vi "resize U16 2D img (SubVI).vi"(7 "Interpolation Type":u32(ring)=1 items=["Zero Order", "Bi-Linear", "Quadratic", "Cubic Spline"], 8 "IMAQ(T)/1D-indexing(1F)":bool=TRUE, 9 "Y Resolution":i32, 10 "X Resolution":i32, 11 "Array":u16[][](array[numeric])) -> (3 "Image Pixels (U16)":u16[][](array[numeric]))   [LabVIEW 2024]
uses:
  <vilib>/vision/NI_Vision_Development_Module.lvlib
panel:
  out "time":dbl
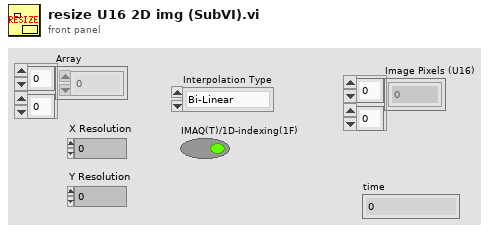
[diagram p1: front panel]
types:
  T1 = typedef "Image Type" = u32
  T2 = typedef "IMAQ Image.ctl" = refnum<image>
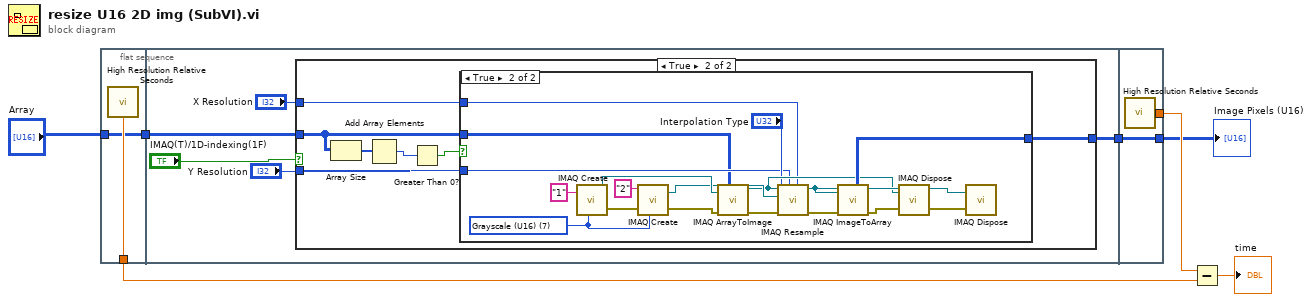
[diagram p0: block diagram]
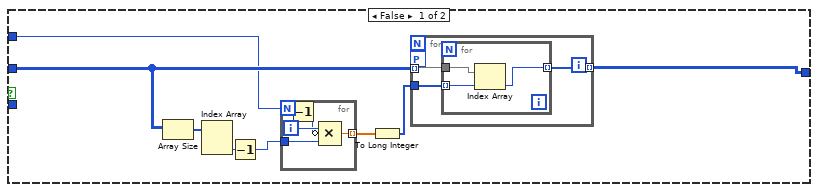
[diagram p2: hidden frame]
diagram:
  n1 = flat-sequence {
    tunnel: [w9] -> w6
    tunnel: [w8] -> w5
    tunnel: "Array" -> [w8]
    tunnel: w5 -> [w13]
    tunnel: [w14] -> w2
    tunnel: [w61] -> w7
    tunnel: [w60] -> w3
    tunnel: w2 -> [w60]
    frame #0 {
      n2 = call <vilib>:"High Resolution Relative Seconds.vi"() -> ("relative seconds"=w9:dbl)
    }
    frame #1 {
      n3 = case shown="True" "IMAQ(T)/1D-indexing(1F)" {
        tunnel: [w22 w40] -> w14
        tunnel: w13 -> [w21 w35]
        tunnel: "X Resolution" -> [w15 w39]
        tunnel: "Y Resolution" -> [_ w38]
        frame False {
          n4 = Array Size(array=w21) -> (size(s)=w20:i32[])
          n5 = Index Array(array=w20) -> (element #2=w19:i32)  [unwired: 2 in, 1 out]
          n6 = Decrement(x=w19) -> (x-1=w17:i32)
          n7 = for {
            N: w15 -> [w25]
            tunnel: w17 -> [w26]
            tunnel: [w24] -> w18 mode=indexing
            i -> [w27]
            n8 = Decrement(x=w25) -> (x-1=w23:i32)
            n9 = Compound Arithmetic op=MULTIPLY(w27, invert w23, w26) -> (w24:dbl)
          }
          n10 = To Long Integer(number=w18) -> (32bit integer=w16:i32[])
          n11 = for {
            tunnel: w21 -> [w30] mode=indexing
            tunnel: [w29] -> w22 mode=indexing
            tunnel: w16 -> [w28]
            workers-P: _ -> [_]
            n12 = for {
              tunnel: w30 -> [w33]
              tunnel: [w32] -> w29 mode=indexing
              tunnel: w28 -> [w31] mode=indexing
              n13 = Index Array(array=w33, index=w31) -> (element=w32:u16)
            }
          }
        }
        frame True {
          n14 = Array Size(array=w35) -> (size(s)=w36:i32[])
          n15 = Add Array Elements(numeric array=w36) -> (sum=w37:i32)
          n16 = Greater Than 0?(x=w37) -> (x > 0?=w34:bool)
          n17 = case shown="True" w34 {
            tunnel: [w41 w49] -> w40
            tunnel: w39 -> [_ w44]
            tunnel: w38 -> [_ w43]
            tunnel: w35 -> [w41 w42]
            frame False {
            }
            frame True {
              w46 = T1 7 items=["Grayscale (U8)", "Grayscale (I16)", "Grayscale (SGL)", "Complex (CSG)", "RGB (U32)", "HSL (U32)", "RGB (U64)", "Grayscale (U16)"] ("Image Type")
              n18 = call "IMAQ Create"("Image Name"="1", "Image Type"=w46) -> ("New Image"=w51:T2, "error out"=w59:errorcluster)  [unwired: 3 in]
              n19 = call "IMAQ Create"("Image Name"="2", "Image Type"=w46, "error in (no error)"=w59) -> ("New Image"=w50:T2, "error out"=w58:errorcluster)  [unwired: 2 in]
              n20 = call "IMAQ ArrayToImage"("Image Pixels (U16)"=w42, "error in (no error)"=w58, "Image"=w51) -> ("error out"=w57:errorcluster, "Image Out"=w47:T2)  [unwired: 7 in]
              n21 = call "IMAQ Resample"("X Resolution"=w44, "Y Resolution"=w43, "error in (no error)"=w57, "Interpolation Type"="Interpolation Type", "Image Dst"=w50, "Image Src"=w47) -> ("error out"=w56:errorcluster, "Image Dst Out"=w48:T2)  [unwired: 4 in]
              n22 = call "IMAQ ImageToArray"("error in (no error)"=w56, "Image"=w48) -> ("Image Pixels (U16)"=w49:u16[][], "error out"=w55:errorcluster)  [unwired: 2 in, 3 out]
              n23 = call "IMAQ Dispose"("Image"=w47, "error in (no error)"=w55) -> ("error out"=w54:errorcluster)  [unwired: 4 in]
              n24 = call "IMAQ Dispose"("Image"=w48, "error in (no error)"=w54) -> ()  [unwired: 4 in, 1 out]
            }
          }
        }
      }
    }
    frame #2 {
      n25 = call <vilib>:"High Resolution Relative Seconds.vi"() -> ("relative seconds"=w61:dbl)
    }
  }
  n26 = Subtract(x=w7, y=w6) -> (x-y=→"time":dbl)
  "Image Pixels (U16)" <- w3
